vi "Error conexión.vi"(8 "error in (no error)":errorcluster, 11 "VISA Refnum in":refnum<visa-resource-name>) -> (2 "Fallo en conexion":bool, 3 "VISA Refnum out":refnum<visa-resource-name>)   [LabVIEW 2020, in "UI Actor.lvlib" / "UI Actor.lvclass"]
uses:
  UI Actor.lvclass
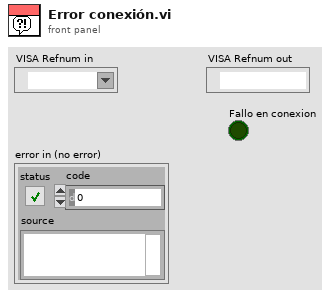
[diagram p1: front panel]
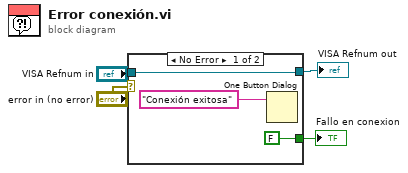
[diagram p0: block diagram]
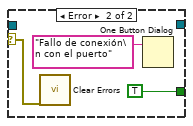
[diagram p2: hidden frame]
diagram:
  n1 = case shown="No Error" "error in (no error)" {
    selector: "error in (no error)" -> [_ w9]
    tunnel: [w6 _] -> w4
    tunnel: "VISA Refnum in" -> [w6 _]
    tunnel: [FALSE TRUE] -> w1
    frame No Error {
      n2 = One Button Dialog(message="Conexión exitosa") -> ()  [unwired: 1 in, 1 out]
    }
    frame Error {
      n3 = call <vilib>:"Clear Errors.vi"("error in (no error)"=w9) -> ()  [unwired: 5 in, 2 out]
      n4 = One Button Dialog(message="Fallo de conexión\n con el puerto") -> ()  [unwired: 1 in, 1 out]
    }
  }
  "VISA Refnum out" <- w4
  "Fallo en conexion" <- w1
